vi "Write Array - Numeric.vi"(8 "error in (no error)":errorcluster, 10 "Array - Numeric":dbl[](array[numeric]), 11 "TAS_Message in":refnum<class "TAS_Message.lvclass">) -> (0 "error out":errorcluster, 3 "TAS_Message out":refnum<class "TAS_Message.lvclass">)   [LabVIEW 2012, in "TAS_Message.lvclass"]
uses:
  TAS_Message.lvclass
  TAS_Message.lvclass/TAS_Message.ctl
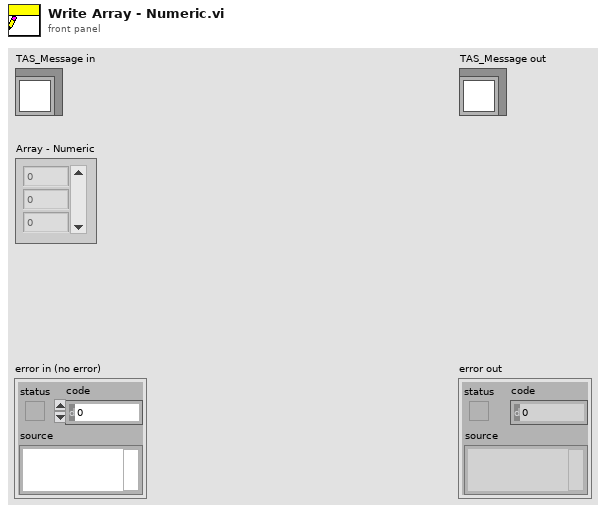
[diagram p1: front panel]
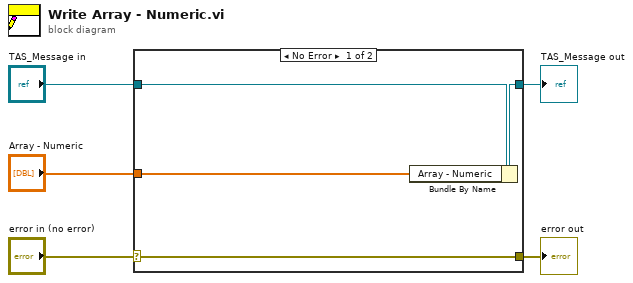
[diagram p0: block diagram]
diagram:
  n1 = case shown="No Error" "error in (no error)" {
    selector: "error in (no error)" -> [w9 w10]
    tunnel: [w9 w10] -> w4
    tunnel: [w7 w11] -> w2
    tunnel: "TAS_Message in" -> [w8 w11]
    tunnel: "Array - Numeric" -> [w6 _]
    frame No Error {
      n2 = Bundle By Name(cluster=w8, "Array - Numeric"=w6) -> (w7:refnum<class "TAS_Message.lvclass">)
    }
    frame Error {
    }
  }
  "error out" <- w4
  "TAS_Message out" <- w2
